vi "CThread Base - Is Run Completed.vi"(5 "RefIn":i32) -> (6 "Completed?":bool)   [LabVIEW 2012, in "CThread.lvlib"]
uses:
  CThread.lvlib
  CRef/CRef.lvlib
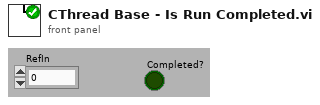
[diagram p1: front panel]
types:
  T1 = typedef "CRef.lvlib/Boolean CReference.ctl" = cluster{"Boolean CRef Address":u16, "Type":enum8{"Null", "Boolean", "U8", "I8", "U16", "I16", "U32", "I32", "U64", "I64", "Single", "Double", "Extended", "CSG", "CDB", "CXT", "Boolean(Def)"}}
  T2 = typedef "CRef.lvlib/Variant CReference.ctl" = cluster{"Generic CRef Address":u16, "Type":u8}
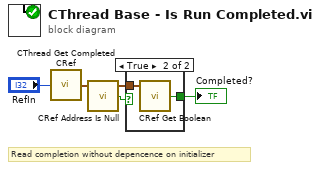
[diagram p0: block diagram]
diagram:
  # "Read completion without depencence on initializer"
  n1 = call "CThread Get Completed CRef.vi"("index"="RefIn") -> ("CRef: Complete?"=w5:T1)  [unwired: 4 in]
  n2 = call "CRef Address Is Null.vi"("Any CReference"=w5) -> ("Null?"=w4:bool, "Variant CReference"=w3:T2)  [unwired: 1 in]
  n3 = case shown="True" w4 {
    tunnel: w3 -> [_ w7]
    tunnel: [_ w6] -> w2
    frame False {
    }
    frame True {
      n4 = call "CRef Get Boolean.vi"("Boolean CReference"=w7) -> ("Value"=w6:bool)  [unwired: 3 in, 1 out]
    }
  }
  "Completed?" <- w2
